vi "SENS_OFFS_STOP.vi"(0 "VISA IN":refnum<visa-resource-name>, 5 "error in":errorcluster, 7 "Channel":i32) -> (14 "VISA Out":refnum<visa-resource-name>, 16 "Data":string, 19 "error out":errorcluster)   [LabVIEW 2018, in "PNA-X.lvlib"]
doc: "SENSe<cnum>:OFFSet:STOP? \n(Read-Only) Returns the response stop frequency. \nParameters \n<cnum> Any existing channel number. If unspecified, value is set to 1 \nExamples SENS:OFFS:STOP \nsense2:offset:stop \nReturn Type Numeric \nDefault Not applicable \n1793\n\nSense:Path:Configuration Commands \nControls the path configuration settings. \nClick on a blue keyword to view the command details. \nSee Also \nExample Programs \nLearn about Path Configuration \nSynchronizing the PNA and Controller \nSCPI Command Tree \nSENSe:PATH:CONFiguration:CATalog? \n(Read-only) Returns a list of configuration names stored in the PNA. \nExamples SENS:PATH:CONF:CAT? \nReturn Type Comma-separated list of double-quoted strings \nDefault Not Applicable \nSENSe:PATH:CONFiguration:DELete <string> \n1794\n\n(Write-only) Deletes the specified configuration name from the PNA. The factory configurations cannot be \ndeleted. This is the only method of distinguishing a factory configuration from a user-named configuration. \nParameters \n<string> Configuration name to be deleted. \nExamples SENS:PATH:CONF:DEL \"MyMixer\" \nReturn Type Not Applicable \nDefault Not Applicable \nSENSe:PATH:CONFiguration:DTEXt <string> \n(Read-Write) Write and read descriptive text associated with the configuration. This text is displayed in the path \nconfiguration dialog. Text is generally used to describe external connections that must be made manually to \ncomplete the configuration setup. \nParameters \n<string> Descriptive text enclosed in quotes. Double quotes are not allowed within the descriptive \ntext. \nExamples SENS:PATH:CONF:DTEX \"Connect J1 jumper on the rear panel.\" \nQuery Syntax SENSe<ch>:PATH:CONFiguration:DTEXt? \nReturn Type String \nDefault Not Applicable \nSENSe<ch>:PATH:CONFiguration:ELEMent:CATalog? \n1795\n\n(Read-only) Returns the names of configurable elements as a comma-delimited list of strings. \nSee a list of configurable elements and settings for various PNA models. \nParameters \n<ch> Any existing channel number; if unspecified, value is set to 1. \nExamples SENS:PATH:CONF:ELEM:CAT? \n'returns \n�Combiner�, �Src1�, �Src2� \nDefault Not Applicable \nSENSe<ch>:PATH:CONFiguration:ELEMent[:STATe] <elem>, <setting> \n(Read-Write) Write or read the setting of a specified element in the current configuration. \nSee a list of configurable elements and settings for various PNA models. \nParameters \n<ch> Any existing channel number; if unspecified, value is set to 1. \n<elem> Name of the element for which a setting is to be made. \n<setting> Element setting. Use SENS:PATH:CONF:ELEM:VAL:CAT? to return a list of valid \nsettings for the specified element. \nExamples SENS:PATH:CONF:ELEM \"Combiner\",\"Normal\" \nQuery Syntax SENSe<ch>:PATH:CONFiguration:ELEMent? \"Combiner\" \nReturns the current state of the Combiner element. \nReturn Type String \nDefault Not applicable \nSENSe<ch>:PATH:CONFiguration:ELEMent:VALue:CATalog? <element> \n1796\n\n(Read-only) Returns the list of valid settings that can be used with the specified element. \nSee a list of configurable elements and settings for various PNA models. \nParameters \n<ch> Any existing channel number; if unspecified, value is set to 1. \n<element> String. Element name for which to return valid settings. \nExamples SENS:PATH:CONF:ELEM:VAL:CAT? \"Combiner\" \n'returns \"Normal\", \"Reversed\" \nDefault Not Applicable \nSENSe<ch>:PATH:CONFiguration:NAME? \n(Read-only) Returns the name of the current configuration only if NO individual element settings had been \nchanged since selecting or storing a configuration. When element settings change, the path configuration name is \ncleared. \nParameters \n<ch> Any existing channel number; if unspecified, value is set to 1. \nExamples SENS:PATH:CONF:NAME? \n'returns \"Default\" \nReturn Type String \nDefault Not Applicable \nSENSe<ch>:PATH:CONFiguration:SELect <string> \n1797\n\n(Write only) Loads the named configuration onto the specified channel. \nUse SENS:PATH:CONF:CAT? to return the configuration names that are stored on the PNA. \nParameters \n<ch> Any existing channel number; if unspecified, value is set to 1. \n<string> Configuration name. \"Default\" is the default factory configuration. \nExamples SENS:PATH:CONF:SEL 'default' \nsense2:path:configuration:select \"MyMixer\" \nQuery Syntax Not Applicable \nDefault \"Default\" \nSENSe<ch>:PATH:CONFiguration:STORe <name> \n(Write only) Saves the path configuration currently associated with channel <ch> to the specified configuration \nname. \nParameters \n<ch> Any existing channel number; if unspecified, value is set to 1. \n<name> String. Configuration name. Factory configurations can NOT be overwritten. Specifying \nthe name of a pre-defined factory configuration will result in an error. \nExamples SENS:PATH:CONF:STOR \"MyMixer\" \nQuery Syntax Not Applicable \nDefault Not Applicable \nLast Modified: \n14-Dec-6 MX New Topic \n1798\n\nSense:Power Command \nLearn about Receiver Attenuation"
uses:
  PNA-X.lvlib
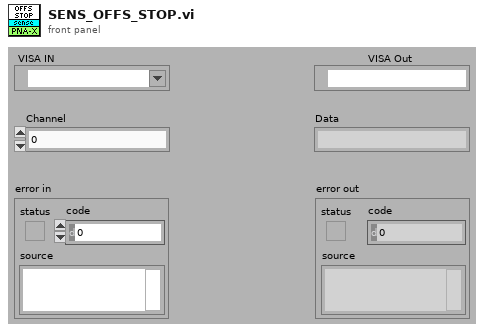
[diagram p1: front panel]
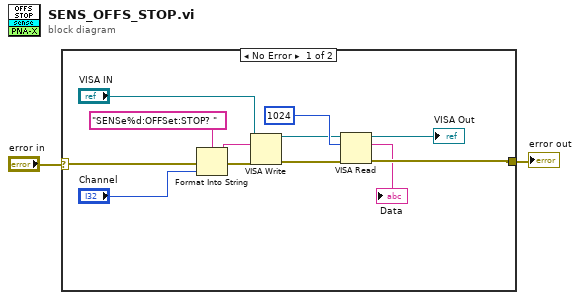
[diagram p0: block diagram]
diagram:
  n1 = case shown="No Error" "error in" {
    selector: "error in" -> [w14 w15]
    tunnel: [w5 w15] -> w1
    frame No Error {
      n2 = Format Into String(format string="SENSe%d:OFFSet:STOP? " ("Cmdline"), error in=w14, "Channel") -> (resulting string=w12:string, error out=w13:errorcluster)  [unwired: 1 in]
      n3 = VISA Write(VISA resource name="VISA IN", write buffer=w12, error in (no error)=w13) -> (VISA resource name out=w7:refnum<visa-resource-name>, error out=w9:errorcluster)  [unwired: 1 out]
      n4 = VISA Read(VISA resource name=w7, byte count=1024, error in (no error)=w9) -> (VISA resource name out=→"VISA Out":refnum<visa-resource-name>, read buffer=→"Data":string, error out=w5:errorcluster)  [unwired: 1 out]
    }
    frame Error {
    }
  }
  "error out" <- w1
